vi "Pre Launch Init.vi"(11 "Nested in":refnum<class "TCP 380.lvclass">) -> (0 "error out":errorcluster, 3 "Nested out":refnum<class "TCP 380.lvclass">)   [LabVIEW 2021, in "TCP 380.lvclass"]
doc: "(<B>Filename</B>: Actor Framework.lvlib:Actor.lvclass:Pre Launch Init.vi)\n\nDefines behavior that occurs after the Launch Nested Actor method is invoked but before the actor's Actor Core method begins running.\n\nBy default, this method does nothing. A descendant class may override it to define behavior."
uses:
  TCP 380.lvclass
  TCP 380.lvclass/TCP 380.ctl
  <vilib>/MGI/Panel Manager/Panel Actor/Panel Actor/Panel Actor.lvclass
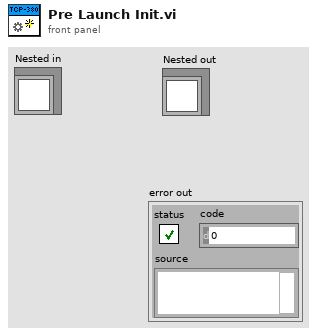
[diagram p1: front panel]
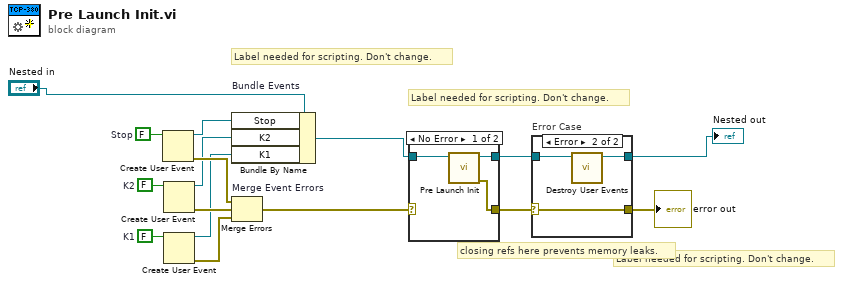
[diagram p0: block diagram]
diagram:
  w5 = FALSE  # K1
  w8 = FALSE  # K2
  w16 = FALSE  # Stop
  # "Label needed for scripting. Don't change."
  # "Label needed for scripting. Don't change."
  # "Label needed for scripting. Don't change."
  # "closing refs here prevents memory leaks."
  n1 = Create User Event(user event datatype=w16) -> (user event=w14:refnum<user-event>, error out=w15:errorcluster)  [unwired: 1 in]
  n2 = Create User Event(user event datatype=w8) -> (user event=w7:refnum<user-event>, error out=w6:errorcluster)  [unwired: 1 in]
  n3 = Create User Event(user event datatype=w5) -> (user event=w4:refnum<user-event>, error out=w3:errorcluster)  [unwired: 1 in]
  n4 = Bundle By Name "Bundle Events"(cluster="Nested in", "Stop"=w14, "K2"=w7, "K1"=w4) -> (w11:refnum<class "TCP 380.lvclass">)
  n5 = Merge Errors "Merge Event Errors"(w15, w6, w3) -> (w10:errorcluster)
  n6 = case shown="No Error" w10 {
    selector: w10 -> [_ w21]
    tunnel: [w19 w20] -> w12
    tunnel: w11 -> [w18 w20]
    tunnel: [w17 w21] -> w9
    frame No Error {
      n7 = call-parent "Pre Launch Init.vi"("Panel Actor in"=w18) -> ("error out"=w17:errorcluster, "Panel Actor out"=w19:refnum<class "TCP 380.lvclass">)  [unwired: 9 in]
    }
    frame Error {
    }
  }
  n8 = case "Error Case" shown="Error" w9 {
    selector: w9 -> [w22 w26]
    tunnel: w12 -> [w23 w25]
    tunnel: [w23 w24] -> w1
    tunnel: [w22 w26] -> w13
    frame No Error {
    }
    frame Error {
      n9 = call "Destroy User Events.vi"("UI Template in"=w25) -> ("UI Template out"=w24:refnum<class "TCP 380.lvclass">)  [unwired: 10 in]
    }
  }
  "error out" <- w13
  "Nested out" <- w1
